vi "Device Params 2 Config INI File.vi"(7 "error in":errorcluster, 8 "Device Connections":T5={"PID Connections"={"Integrator DAQ Channels"={"V0"="cDAQ1Mod1/ai0", "S1"="cDAQ1Mod5/port0/line4", "S2"="cDAQ1Mod5/ctr0"}}}, 9 "Device Settings":T8={"Detector Type"=enum."Photo-Ionization Detector", "MFC Type"=enum."Aalborg GFC17", "PS Type"=enum."Stanford Research PS350", "Detector Connection"=FALSE, "Detector Sampling Frequency"=0.0, "MFC Connection"=FALSE, "MFC Flow Rate"=0.0, "MFC Valve Status"=enum."Open", "PS Connection"=FALSE, "PS Source Mode"=enum."Volts", "PS Source Value"=0.0, "PS Source Value Units"=enum."volts", "Limits"={"Voltage Limit"=0.0, "Voltage Limit Units"=enum."volts", "Current Limit"=0.0, "Current Limit Units"=enum."amps", "Voltage Trip/Cmpl"=0.0, "Voltage Trip/Cmpl Units"=enum."volts", "Current Trip/Cmpl"=0.0, "Current Trip/Cmpl Units"=enum."amps"}, "PID Integration Time"=10.0, "PID Grid Voltage"=10.0, "Valve Type"=enum."SMC - INL Controller", "Valve Assembly"={"Valve 1"=FALSE, "Valve 2"=FALSE, "Valve 3"=FALSE, "Valve 4"=FALSE, "Valve 5"=FALSE}, "Valve Connection"=FALSE}, 10 "Configuration in":refnum<class "Configuration.lvclass">) -> (0 "error out":errorcluster, 3 "Configuration out":refnum<class "Configuration.lvclass">)   [LabVIEW 2011]
uses:
  Modules/File/Configuration/Configuration.lvclass
  Controls/Device Settings.ctl
  Modules/Hardware/Mass Flow Controller/Valve Status.ctl
  Modules/Hardware/Power Supply/Source Mode.ctl
  Modules/Hardware/Power Supply/Source Units.ctl
  Modules/Hardware/Power Supply/Protection Limits.ctl
  Modules/Hardware/Power Supply/Voltage Units.ctl
  Modules/Hardware/Power Supply/Current Units.ctl
  Controls/Valve Type.ctl
  Modules/Hardware/Valve Controller/Valve Assembly.ctl
  Controls/Device Connections.ctl
  Modules/Hardware/PID/PID Connections.ctl
  Modules/Hardware/PID/Integrator DAQmx Channels.ctl
  Modules/File/Configuration/PID Keys.ctl
  Modules/File/Configuration/PID Key Types.ctl
  Modules/File/Configuration/Key Data Type.ctl
  Modules/File/Configuration/PID Sections.ctl
  Modules/Hardware/Power Supply/Power Supply.lvclass
  Modules/Hardware/Mass Flow Controller/Mass Flow Controller.lvclass
  Modules/Hardware/PID/PID.lvclass
  Modules/Hardware/Valve Controller/Valve Controller.lvclass
panel:
  in  "Sections":T1=["Devices", "Devices", "Devices", "Devices", "Devices", "Devices", "Devices", "Devices", "Devices", "Devices", "Devices", "Devices", "Devices", "Devices", "Devices", "Devices", "Devices", "Devices", "Devices", "Devices", "Devices", "Devices", "Device Connections", "Device Connections", "Device Connections"]
  in  "Key Types":T2=[enum."I32", enum."I32", enum."I32", enum."I32", enum."I32", enum."I32", enum."I32", enum."I32", enum."I32", enum."I32", enum."Double", enum."Double", enum."Double", enum."Double", enum."Double", enum."Double", enum."Double", enum."Double", enum."Double", enum."Boolean", enum."Boolean", enum."Boolean", enum."DAQmx Channel", enum."DAQmx Channel", enum."DAQmx Channel"]
  in  "Keys":T4=["Detector type", "MFC Type", "PS Type", "PS Source Units", "PS Source Mode", "MFC Valve Status", "PS Voltage Limit Units", "PS Current Limit Units", "PS Voltage Trip/Cmpl Units", "PS Current Trip/Cmpl Units", "PS Source Value", "MFC Flow Rate", "Detector Sampling Frequency", "PS Voltage Limit", "PS Current Limit", "PS Voltage Trip/Cmpl", "PS Current Trip/Cmpl", "PID Grid Voltage", "PID Integration Time", "Detector Connection", "MFC Connection", "PS Connection", "PID Integrator DAQmx Channel V0", "PID Integrator DAQmx Channel S1", "PID Integrator DAQmx Channel S2"]
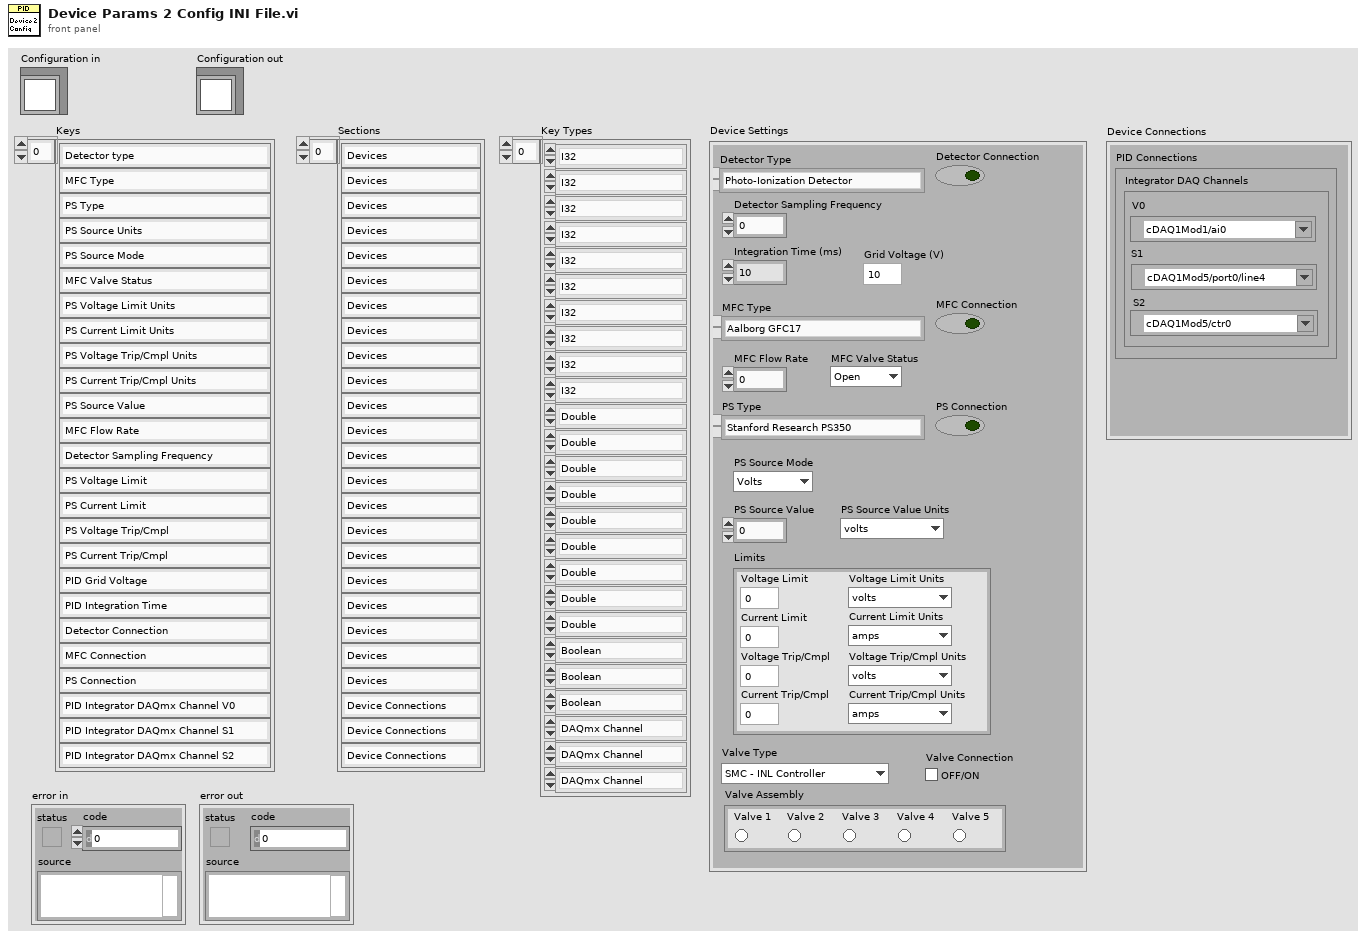
[diagram p1: front panel]
types:
  T1 = typedef "Configuration.lvclass/PID Sections.ctl" = string[]
  T2 = typedef "Configuration.lvclass/PID Key Types.ctl" = T3[]
  T3 = typedef "Configuration.lvclass/Key Data Type.ctl" = enum16{"Boolean", "U32", "I32", "Double", "String", "DAQmx Channel", "Path"}
  T4 = typedef "Configuration.lvclass/PID Keys.ctl" = string[]
  T5 = typedef "Device Connections.ctl" = cluster{"PID Connections":T6}
  T6 = typedef "PID.lvclass/PID Connections.ctl" = cluster{"Integrator DAQ Channels":T7}
  T7 = typedef "PID.lvclass/Integrator DAQmx Channels.ctl" = cluster{"V0":tag, "S1":tag, "S2":tag}
  T8 = typedef "Device Settings.ctl" = cluster{"Detector Type":enum16{"Photo-Ionization Detector"}, "MFC Type":enum16{"Aalborg GFC17"}, "PS Type":enum16{"Stanford Research PS350", "Keithley 2400"}, "Detector Connection":bool, "Detector Sampling Frequency":dbl, "MFC Connection":bool, "MFC Flow Rate":dbl, "MFC Valve Status":T9, "PS Connection":bool, "PS Source Mode":T10, "PS Source Value":dbl, "PS Source Value Units":T11, "Limits":T12, "PID Integration Time":dbl, "PID Grid Voltage":dbl, "Valve Type":T15, "Valve Assembly":T16, "Valve Connection":bool}
  T9 = typedef "Mass Flow Controller.lvclass/Valve Status.ctl" = enum16{"Open", "Closed"}
  T10 = typedef "Power Supply.lvclass/Source Mode.ctl" = enum16{"Volts", "Current"}
  T11 = typedef "Power Supply.lvclass/Source Units.ctl" = enum16{"volts", "millivolts", "microvolts", "amps", "milliamps", "microamps", "nanoamps"}
  T12 = typedef "Power Supply.lvclass/Protection Limits.ctl" = cluster{"Voltage Limit":dbl, "Voltage Limit Units":T13, "Current Limit":dbl, "Current Limit Units":T14, "Voltage Trip/Cmpl":dbl, "Voltage Trip/Cmpl Units":T13, "Current Trip/Cmpl":dbl, "Current Trip/Cmpl Units":T14}
  T13 = typedef "Power Supply.lvclass/Voltage Units.ctl" = enum16{"volts", "millivolts", "microvolts"}
  T14 = typedef "Power Supply.lvclass/Current Units.ctl" = enum16{"amps", "milliamps", "microamps", "nanoamps"}
  T15 = typedef "Valve Type.ctl" = enum16{"SMC - INL Controller"}
  T16 = typedef "Valve Controller.lvclass/Valve Assembly.ctl" = cluster{"Valve 1":bool, "Valve 2":bool, "Valve 3":bool, "Valve 4":bool, "Valve 5":bool}
  T17 = enum16{"Stanford Research PS350", "Keithley 2400"}
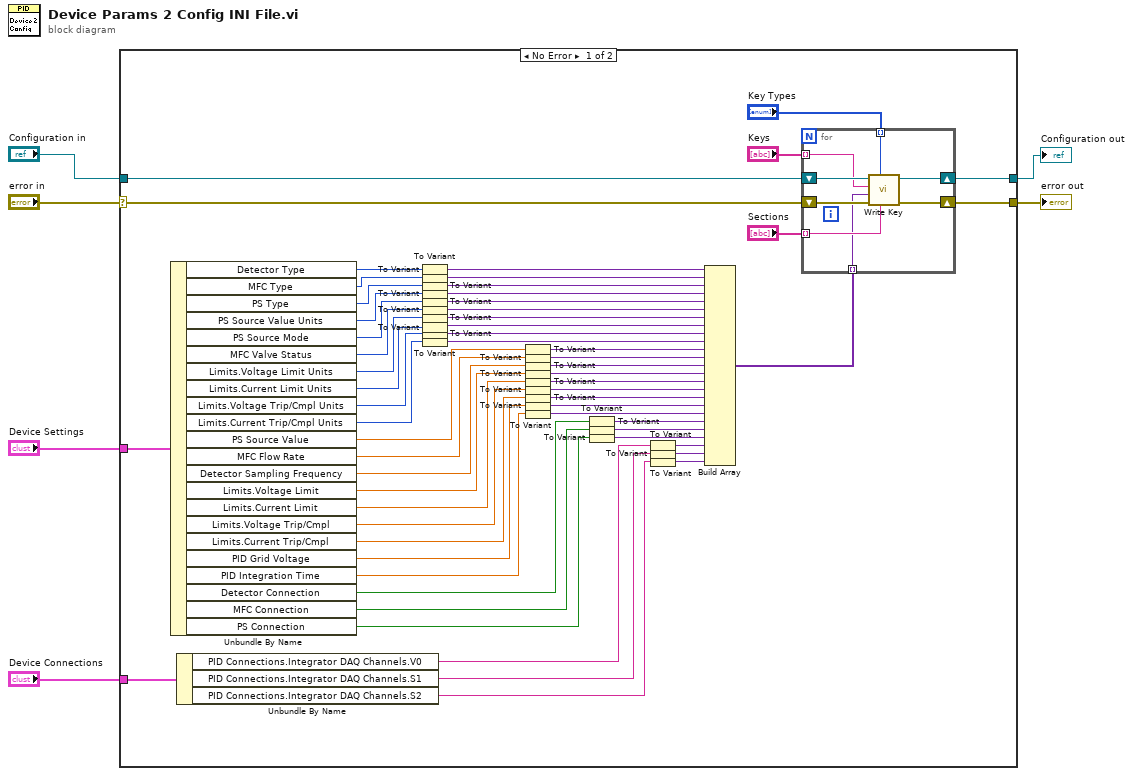
[diagram p0: block diagram]
diagram:
  n1 = case shown="No Error" "error in" {
    selector: "error in" -> [w66 w75]
    tunnel: [w8 w76] -> w6
    tunnel: "Configuration in" -> [w65 w76]
    tunnel: [w7 w75] -> w4
    tunnel: "Device Settings" -> [w60 _]
    tunnel: "Device Connections" -> [w64 _]
    frame No Error {
      n2 = Unbundle By Name(w60) -> ("Detector Type"=w58:enum16{"Photo-Ionization Detector"}, "MFC Type"=w57:enum16{"Aalborg GFC17"}, "PS Type"=w56:T17, "PS Source Value Units"=w55:T11, "PS Source Mode"=w54:T10, "MFC Valve Status"=w53:T9, "Limits.Voltage Limit Units"=w52:T13, "Limits.Current Limit Units"=w51:T14, "Limits.Voltage Trip/Cmpl Units"=w50:T13, "Limits.Current Trip/Cmpl Units"=w49:T14, "PS Source Value"=w39:dbl, "MFC Flow Rate"=w38:dbl, "Detector Sampling Frequency"=w37:dbl, "Limits.Voltage Limit"=w33:dbl, "Limits.Current Limit"=w32:dbl, "Limits.Voltage Trip/Cmpl"=w31:dbl, "Limits.Current Trip/Cmpl"=w30:dbl, "PID Grid Voltage"=w29:dbl, "PID Integration Time"=w28:dbl, "Detector Connection"=w21:bool, "MFC Connection"=w20:bool, "PS Connection"=w19:bool)
      n3 = Unbundle By Name(w64) -> ("PID Connections.Integrator DAQ Channels.V0"=w15:tag, "PID Connections.Integrator DAQ Channels.S1"=w13:tag, "PID Connections.Integrator DAQ Channels.S2"=w10:tag)
      n4 = To Variant(anything=w58) -> (Variant=w59:variant)
      n5 = To Variant(anything=w57) -> (Variant=w48:variant)
      n6 = To Variant(anything=w56) -> (Variant=w47:variant)
      n7 = To Variant(anything=w55) -> (Variant=w46:variant)
      n8 = To Variant(anything=w54) -> (Variant=w45:variant)
      n9 = To Variant(anything=w53) -> (Variant=w44:variant)
      n10 = To Variant(anything=w52) -> (Variant=w43:variant)
      n11 = To Variant(anything=w51) -> (Variant=w42:variant)
      n12 = To Variant(anything=w50) -> (Variant=w41:variant)
      n13 = To Variant(anything=w49) -> (Variant=w40:variant)
      n14 = To Variant(anything=w39) -> (Variant=w36:variant)
      n15 = To Variant(anything=w38) -> (Variant=w35:variant)
      n16 = To Variant(anything=w37) -> (Variant=w34:variant)
      n17 = To Variant(anything=w33) -> (Variant=w27:variant)
      n18 = To Variant(anything=w32) -> (Variant=w26:variant)
      n19 = To Variant(anything=w31) -> (Variant=w25:variant)
      n20 = To Variant(anything=w30) -> (Variant=w24:variant)
      n21 = To Variant(anything=w29) -> (Variant=w23:variant)
      n22 = To Variant(anything=w28) -> (Variant=w22:variant)
      n23 = To Variant(anything=w21) -> (Variant=w18:variant)
      n24 = To Variant(anything=w20) -> (Variant=w17:variant)
      n25 = To Variant(anything=w19) -> (Variant=w16:variant)
      n26 = To Variant(anything=w15) -> (Variant=w14:variant)
      n27 = To Variant(anything=w13) -> (Variant=w12:variant)
      n28 = To Variant(anything=w10) -> (Variant=w11:variant)
      n29 = Build Array(w59, w48, w47, w46, w45, w44, w43, w42, w41, w40, w36, w35, w34, w27, w26, w25, w24, w23, w22, w18, w17, w16, w14, w12, w11) -> (w9:variant[])
      n30 = for {
        shift-right: [w72] -> w8
        shift-left: w65 -> [w73]
        shift-right: [w71] -> w7
        shift-left: w66 -> [w74]
        tunnel: "Sections" -> [w70] mode=indexing
        tunnel: "Key Types" -> [w69] mode=indexing
        tunnel: "Keys" -> [w68] mode=indexing
        tunnel: w9 -> [w67] mode=indexing
        n31 = call-dynamic "Write Key.vi"("section"=w70, "data type"=w69, "error in (no error)"=w74, "key"=w67, "name"=w68, "Configuration.lvclass in"=w73) -> ("error out"=w71:errorcluster, "Configuration.lvclass out"=w72:refnum<class "Configuration.lvclass">)  [unwired: 4 in]
      }
    }
    frame Error {
    }
  }
  "Configuration out" <- w6
  "error out" <- w4
